vi "pareseXML_AcqInfo.vi"(8 "error in (no error)":errorcluster, 11 "Raw Package without Header":string) -> (0 "error out":errorcluster, 3 "AcquisitionInfo":T1)   [LabVIEW 2020, in "OXYGEN_Datastream.lvlib"]
uses:
  OXYGEN_Datastream.lvlib
  TypeDefs/AcqInfo_AcquisitionStart.ctl
  TypeDefs/AcqInfo_AcquisitionStart_nanoseconds.ctl
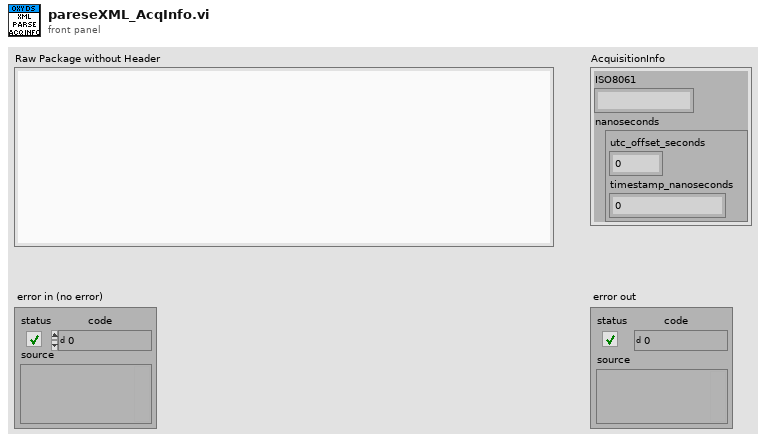
[diagram p1: front panel]
types:
  T1 = typedef "OXYGEN_Datastream.lvlib/AcqInfo_AcquisitionStart.ctl" = cluster{"ISO8061":string, "nanoseconds":T2}
  T2 = typedef "OXYGEN_Datastream.lvlib/AcqInfo_AcquisitionStart_nanoseconds.ctl" = cluster{"utc_offset_seconds":i64, "timestamp_nanoseconds":i64}
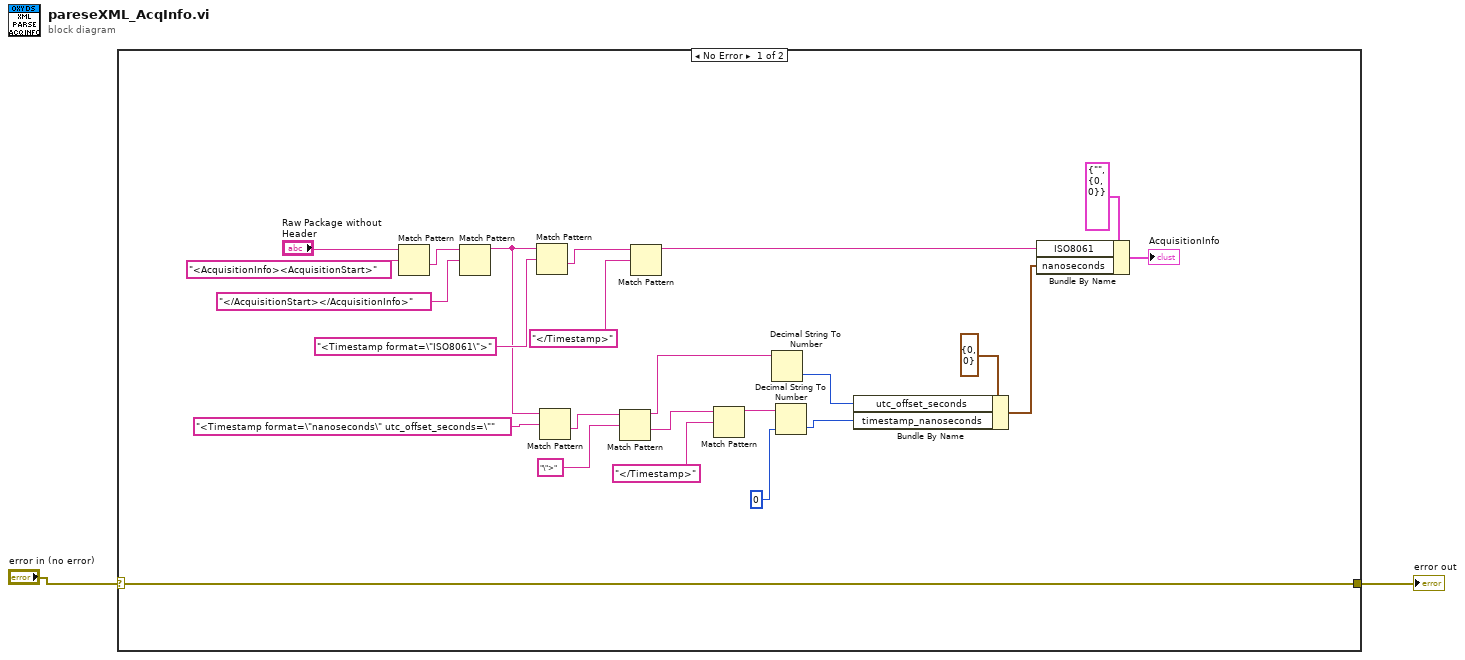
[diagram p0: block diagram]
diagram:
  n1 = case shown="No Error" "error in (no error)" {
    selector: "error in (no error)" -> [w3 w27]
    tunnel: [w3 w27] -> w1
    frame No Error {
      n2 = Match Pattern(string="Raw Package without Header", regular expression="<AcquisitionInfo><AcquisitionStart>") -> (after substring=w24:string)  [unwired: 1 in, 3 out]
      n3 = Match Pattern(string=w24, regular expression="</AcquisitionStart></AcquisitionInfo>") -> (before substring=w4:string)  [unwired: 1 in, 3 out]
      n4 = Match Pattern(string=w4, regular expression="<Timestamp format=\"ISO8061\">") -> (after substring=w21:string)  [unwired: 1 in, 3 out]
      n5 = Match Pattern(string=w4, regular expression="<Timestamp format=\"nanoseconds\" utc_offset_seconds=\"") -> (after substring=w15:string)  [unwired: 1 in, 3 out]
      n6 = Match Pattern(string=w15, regular expression="\">") -> (before substring=w10:string, after substring=w12:string)  [unwired: 1 in, 2 out]
      n7 = Match Pattern(string=w21, regular expression="</Timestamp>") -> (before substring=w17:string)  [unwired: 1 in, 3 out]
      n8 = Match Pattern(string=w12, regular expression="</Timestamp>") -> (before substring=w6:string)  [unwired: 1 in, 3 out]
      n9 = Decimal String To Number(string=w10) -> (number=w8:i32)  [unwired: 2 in, 1 out]
      n10 = Decimal String To Number(string=w6, default (0L)=i64 0 ("default (0 I32)")) -> (number=w7:i64)  [unwired: 1 in, 1 out]
      n11 = Bundle By Name(cluster=T2 {"utc_offset_seconds"=0, "timestamp_nanoseconds"=0} ("nanoseconds"), "utc_offset_seconds"=w8, "timestamp_nanoseconds"=w7) -> (w11:T2)
      n12 = Bundle By Name(cluster=T1 {"ISO8061"="", "nanoseconds"={"utc_offset_seconds"=0, "timestamp_nanoseconds"=0}} ("AcquisitionStart"), "ISO8061"=w17, "nanoseconds"=w11) -> (→"AcquisitionInfo":T1)
    }
    frame Error {
    }
  }
  "error out" <- w1
